vi "Update.vi"(8 "error in (no error)":errorcluster, 11 "Level Controller in":refnum<class "Level Controller.lvclass">) -> (0 "error out":errorcluster, 3 "Level Controller out":refnum<class "Level Controller.lvclass">)   [LabVIEW 2012, in "Level Controller.lvlib" / "Level Controller.lvclass"]
uses:
  Level Controller.lvclass
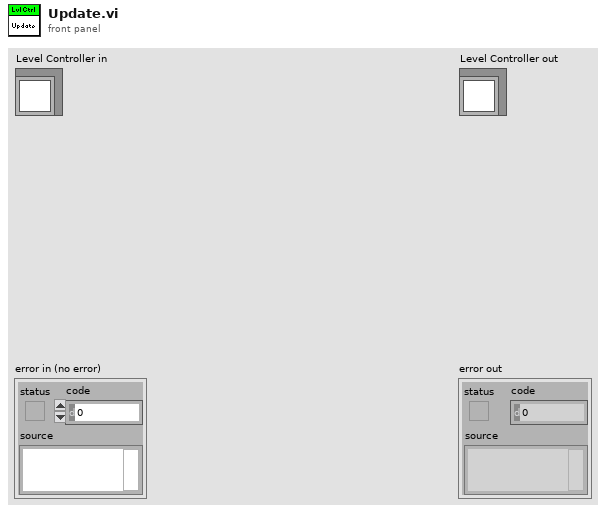
[diagram p1: front panel]
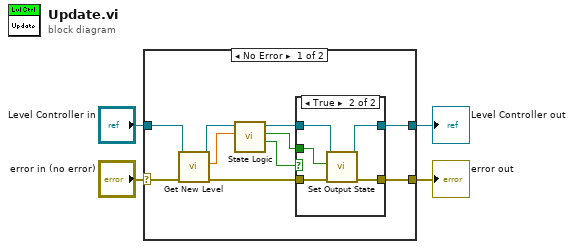
[diagram p0: block diagram]
diagram:
  n1 = case shown="No Error" "error in (no error)" {
    selector: "error in (no error)" -> [w14 w23]
    tunnel: [w13 w23] -> w3
    tunnel: [w10 w22] -> w1
    tunnel: "Level Controller in" -> [w11 w22]
    frame No Error {
      n2 = call-dynamic "Get New Level.vi"("error in (no error)"=w14, "Level Controller in"=w11) -> ("error out"=w12:errorcluster, "Level"=w8:dbl, "Level Controller out"=w9:refnum<class "Level Controller.lvclass">)  [unwired: 7 in]
      n3 = call "State Logic.vi"("Level"=w8, "Level Controller in"=w9) -> ("Changed?"=w5:bool, "Output State"=w6:bool, "Level Controller out"=w7:refnum<class "Level Controller.lvclass">)  [unwired: 7 in]
      n4 = case shown="True" w5 {
        tunnel: [w15 w21] -> w13
        tunnel: w12 -> [w15 w20]
        tunnel: w7 -> [w16 w19]
        tunnel: [w16 w18] -> w10
        tunnel: w6 -> [_ w17]
        frame False {
        }
        frame True {
          n5 = call-dynamic "Set Output State.vi"("error in (no error)"=w20, "Output State"=w17, "Level Controller in"=w19) -> ("error out"=w21:errorcluster, "Level Controller out"=w18:refnum<class "Level Controller.lvclass">)  [unwired: 7 in]
        }
      }
    }
    frame Error {
    }
  }
  "error out" <- w3
  "Level Controller out" <- w1
